vi "Asylum_WriteString.vi"(8 "error in (no error)":errorcluster, 9 "valueString":string, 10 "parameterName":string, 11 "Application":refnum<k7>) -> (0 "error out":errorcluster, 3 "Application":refnum<k7>)   [LabVIEW 2019]
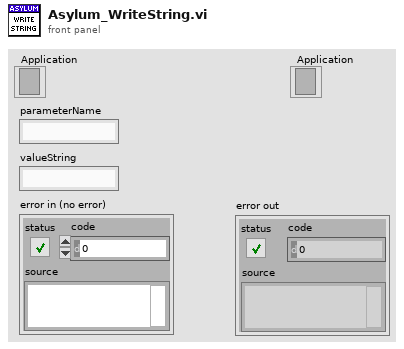
[diagram p1: front panel]
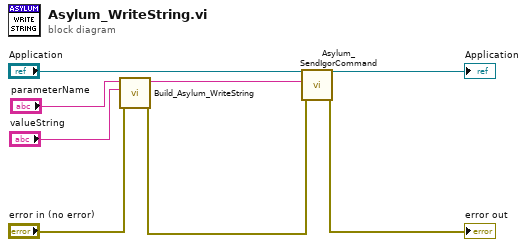
[diagram p0: block diagram]
diagram:
  n1 = call "Build_Asylum_WriteString.vi"("error in (no error)"="error in (no error)", "valueString"="valueString", "parameterName"="parameterName") -> ("error out"=w2:errorcluster, "String"=w8:string)  [unwired: 7 in]
  n2 = call "Asylum_SendIgorCommand.vi"("error in (no error)"=w2, "command"=w8, "Application In"="Application") -> ("error out"=→"error out":errorcluster, "Application Out"=→"Application":refnum<k7>)  [unwired: 5 in, 2 out]
